vi "SetSettings.vi"(8 "error in (no error)":errorcluster, 10 "Variant":variant, 11 "PacificPowerSource in":refnum<class "PacificPowerSource.lvclass">) -> (0 "error out":errorcluster, 3 "PacificPowerSource Out":refnum<class "PacificPowerSource.lvclass">)   [LabVIEW 2018, in "AcPwrPlugins.lvlib" / "PacificPowerSource.lvclass"]
doc: "This VI retrieves a boolean status to see if the instrument can conduct measurements while the device is changing modes or turning off and on."
uses:
  PacificPowerSource.lvclass
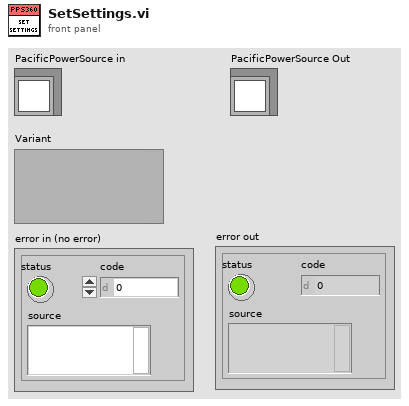
[diagram p1: front panel]
types:
  T1 = typedef "AcPwrPlugins.lvlib/PacificPowerSource.lvclass/Device(s)Settings.ctl" = cluster{"MeasName":string, "Modules":cluster{"Handle":string, "Connected":bool, "Clear Device (F)":bool, "btnIdQuery":bool, "btnReset":bool, "Program #":cluster{"Phase B (Degrees)":i32, "Waveform A (1: Sine)":i32, "Voltage Level (Va)":dbl, "Program Number (0)":i32, "Voltage Level (Vb) ":dbl, "Form (3: Three)":u16, "Coupling  (0: Direct)":u16, "Frequency (45Hz)":dbl, "Current Limit (40A)":dbl, "Phase C (Degrees)":i32, "Voltage Level (Vc)":dbl, "Waveform B (1: Sine)":i32, "Waveform C (1: Sine)":i32}[], "Impedance Parameters (off, 0.00)":cluster{"State":bool, "Impedance":dbl}, "Transient Execution (F)":bool, "OutputEnabled":bool, "Source Range":cluster{"Frequency Minimum (45 Hz)":dbl, "Frequency Maximum (1200 Hz)":dbl, "Voltage Maximum (V)":dbl, "Voltage Minimum (V)":dbl, "Range Control (0: Auto)":u16, "Initial Voltage (0V)":u16, "Frequency Range (600Hz)":u16}, "Port Type":enum16{"GPIB", "Serial"}}[]}
  T2 = typedef "AcPwrPlugins.lvlib/PacificPowerSource.lvclass/Measurements.ctl" = cluster{"Handle":string, "Name":string, "Enabled ":bool, "Measurement Value":dbl, "Channel Name":enum16{"A", "B", "C"}, "Measurement Type ":T3}[]
  T3 = typedef "AcPwrPlugins.lvlib/PacificPowerSource.lvclass/MeasurementType.ctl" = enum16{"Voltage RMS L-N", "Voltage RMS L-L", "Frequency", "Current RMS", "Current Peak", "Crest Factor", "Power Factor", "Power VA", "Real Power"}
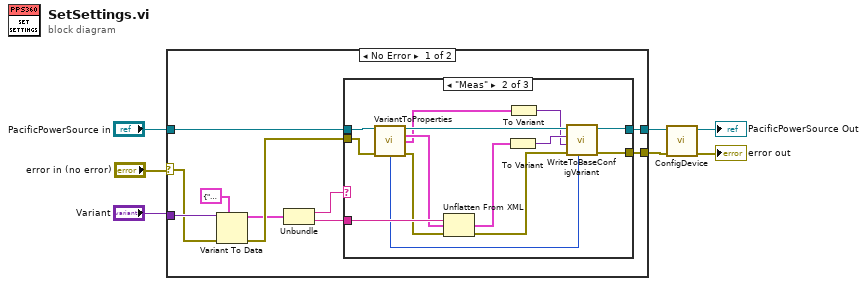
[diagram p0: block diagram]
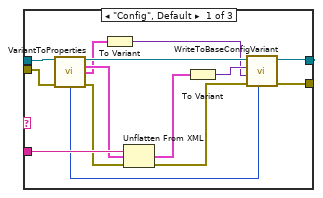
[diagram p2: hidden frame]
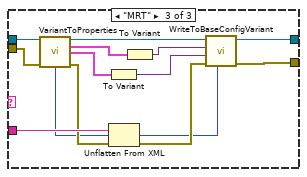
[diagram p3: hidden frame]
diagram:
  n1 = case shown="No Error" "error in (no error)" {
    selector: "error in (no error)" -> [w13 w61]
    tunnel: [w16 w61] -> w4
    tunnel: "PacificPowerSource in" -> [w17 w60]
    tunnel: "Variant" -> [w14 _]
    tunnel: [w15 w60] -> w2
    frame No Error {
      n2 = Variant To Data(error in=w13, type=cluster{string, string} {"", ""}, Variant=w14) -> (data=w10:cluster{string, string}, error out=w11:errorcluster)
      n3 = Unbundle(w10) -> (w8:string, w9:string)
      n4 = case shown="\"Meas\"" w8 {
        tunnel: [w26 w40 w54] -> w16
        tunnel: w17 -> [w30 w44 w58]
        tunnel: [w28 w42 w56] -> w15
        tunnel: w11 -> [w29 w43 w57]
        tunnel: w9 -> [w31 w45 w59]
        frame "Config", Default {
          n5 = call "VariantToProperties.vi"("PacificPowerSource in"=w30, "error in (no error)"=w29) -> ("PacificPowerSource out"=w27:refnum<class "PacificPowerSource.lvclass">, "Device(s)Settings"=w23:T1, "Measurements"=w19:T2, "Measurement Refresh Time (ms)"=w20:u32, "error out"=w25:errorcluster)  [unwired: 7 in, 2 out]
          n6 = To Variant(anything=w19) -> (Variant=w18:variant)
          n7 = Unflatten From XML(xml string=w31, type=w23, error in (no error)=w25) -> (value=w21:T1, error out=w24:errorcluster)
          n8 = To Variant(anything=w21) -> (Variant=w22:variant)
          n9 = call "WriteToBaseConfigVariant.vi"("Measurement Refresh Time (ms)"=w20, "error in (no error)"=w24, "Meas"=w18, "Config"=w22, "PacificPowerSource in"=w27) -> ("error out"=w26:errorcluster, "PacificPowerSource out"=w28:refnum<class "PacificPowerSource.lvclass">)  [unwired: 5 in]
        }
        frame "Meas" {
          n10 = call "VariantToProperties.vi"("PacificPowerSource in"=w44, "error in (no error)"=w43) -> ("PacificPowerSource out"=w41:refnum<class "PacificPowerSource.lvclass">, "Device(s)Settings"=w37:T1, "Measurements"=w33:T2, "Measurement Refresh Time (ms)"=w34:u32, "error out"=w39:errorcluster)  [unwired: 7 in, 2 out]
          n11 = Unflatten From XML(xml string=w45, type=w37, error in (no error)=w39) -> (value=w35:T1, error out=w38:errorcluster)
          n12 = To Variant(anything=w35) -> (Variant=w36:variant)
          n13 = To Variant(anything=w33) -> (Variant=w32:variant)
          n14 = call "WriteToBaseConfigVariant.vi"("Measurement Refresh Time (ms)"=w34, "error in (no error)"=w38, "Meas"=w32, "Config"=w36, "PacificPowerSource in"=w41) -> ("error out"=w40:errorcluster, "PacificPowerSource out"=w42:refnum<class "PacificPowerSource.lvclass">)  [unwired: 5 in]
        }
        frame "MRT" {
          n15 = call "VariantToProperties.vi"("PacificPowerSource in"=w58, "error in (no error)"=w57) -> ("PacificPowerSource out"=w55:refnum<class "PacificPowerSource.lvclass">, "Device(s)Settings"=w46:T1, "Measurements"=w50:T2, "Measurement Refresh Time (ms)"=w48:u32, "error out"=w53:errorcluster)  [unwired: 7 in, 2 out]
          n16 = To Variant(anything=w50) -> (Variant=w49:variant)
          n17 = Unflatten From XML(xml string=w59, type=w48, error in (no error)=w53) -> (value=w47:u32, error out=w52:errorcluster)
          n18 = To Variant(anything=w46) -> (Variant=w51:variant)
          n19 = call "WriteToBaseConfigVariant.vi"("Measurement Refresh Time (ms)"=w47, "error in (no error)"=w52, "Meas"=w49, "Config"=w51, "PacificPowerSource in"=w55) -> ("error out"=w54:errorcluster, "PacificPowerSource out"=w56:refnum<class "PacificPowerSource.lvclass">)  [unwired: 5 in]
        }
      }
    }
    frame Error {
    }
  }
  n20 = call-dynamic "ConfigDevice.vi"("error in (no error)"=w4, "PacificPowerSource in"=w2) -> ("error out"=→"error out":errorcluster, "PacificPowerSource out"=→"PacificPowerSource Out":refnum<class "PacificPowerSource.lvclass">)  [unwired: 8 in]
